vi "practica113b.vi"() -> ()   [LabVIEW 2016]
uses:
  <vilib>/Native 3D Graph/xcontrol/3DPC_SurfacePlot.xctl
panel:
  in  "Sz":dbl(slide) scale=0.0..10.0
  in  "s3":dbl(slide) max=1.4285714285714286 scale=0.0..3.4693877551020407
  in  "xy":dbl(knob) scale=0.0..360.0
  in  "xy2":dbl(knob) scale=-175.0..175.0
  out "3D Graph":refnum<class "Base Datatype.lvclass">[](xcontrol)
  in  "s1":dbl
  in  "s2":dbl
  in  "stop":bool
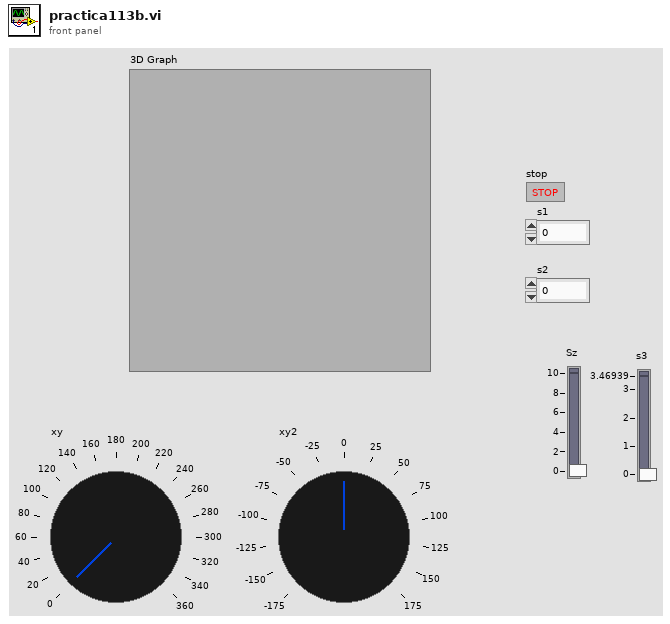
[diagram p1: front panel]
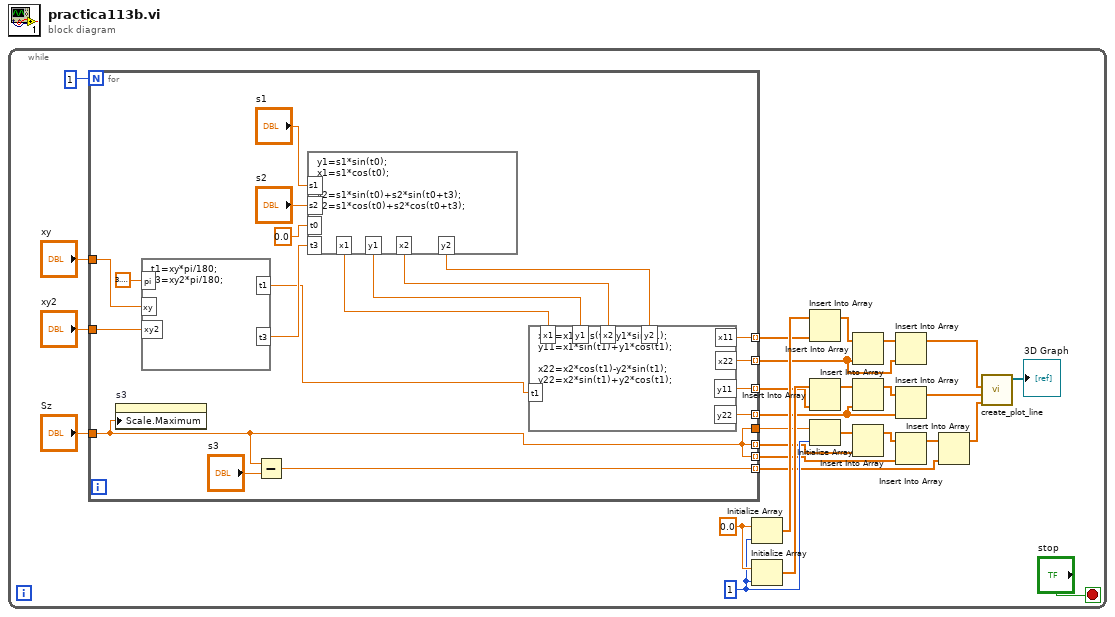
[diagram p0: block diagram]
diagram:
  n1 = while {
    stop <- "stop" stop-if-true
    w18 = 0.0
    w16 = 1 ("dimension size")
    n2 = for {
      N: 1 -> [_]
      tunnel: "xy" -> [w46]
      tunnel: "xy2" -> [w45]
      tunnel: [w33] -> w7 mode=indexing
      tunnel: [w35] -> w17 mode=indexing
      tunnel: [w32] -> w8 mode=indexing
      tunnel: [w34] -> w15 mode=indexing
      tunnel: [w29] -> w14 mode=indexing
      tunnel: [w29] -> w13 mode=indexing
      tunnel: [w30] -> w9 mode=indexing
      tunnel: "Sz" -> [w29]
      tunnel: [w29] -> w1
      n3 = property on="s3" class="Slide (strict)"("Scale.Maximum"=w29) -> ()  [unwired: 2 in, 2 out]
      n4 = formula code="t1=xy*pi/180;\nt3=xy2*pi/180;"("pi"=3.141592653589793, "xy"=w46, "xy2"=w45) -> ("t1"=w38:dbl, "t3"=w43:dbl)
      n5 = Subtract(x=w29, y="s3") -> (x-y=w30:dbl)
      n6 = formula code="y1=s1*sin(t0);\nx1=s1*cos(t0);\n\ny2=s1*sin(t0)+s2*sin(t0+t3);\nx2=s1*cos(t0)+s2*cos(t0+t3);"("t0"=0.0 ("input variable"), "s1"="s1", "s2"="s2", "t3"=w43) -> ("y1"=w39:dbl, "x1"=w40:dbl, "y2"=w36:dbl, "x2"=w37:dbl)
      n7 = formula code="x11=x1*cos(t1)-y1*sin(t1);\ny11=x1*sin(t1)+y1*cos(t1);\n\nx22=x2*cos(t1)-y2*sin(t1);\ny22=x2*sin(t1)+y2*cos(t1);"("x1"=w40, "y1"=w39, "t1"=w38, "x2"=w37, "y2"=w36) -> ("y11"=w34:dbl, "x11"=w35:dbl, "y22"=w32:dbl, "x22"=w33:dbl)
    }
    n8 = Initialize Array(w18, w16) -> (w22:dbl[])
    n9 = Initialize Array(w18, w16) -> (w23:dbl[])
    n10 = Insert Into Array(array=w22, new element=w17) -> (w19:dbl[])  [unwired: 1 in]
    n11 = Insert Into Array(array=w23, new element=w15) -> (w20:dbl[])  [unwired: 1 in]
    n12 = Initialize Array(w1, w16) -> (w3:dbl[])
    n13 = Insert Into Array(array=w19, new element=w7) -> (w12:dbl[])  [unwired: 1 in]
    n14 = Insert Into Array(array=w20, new element=w8) -> (w11:dbl[])  [unwired: 1 in]
    n15 = Insert Into Array(array=w3, new element=w14) -> (w21:dbl[])  [unwired: 1 in]
    n16 = Insert Into Array(array=w12, new element=w7) -> (w6:dbl[])  [unwired: 1 in]
    n17 = Insert Into Array(array=w11, new element=w8) -> (w5:dbl[])  [unwired: 1 in]
    n18 = Insert Into Array(array=w21, new element=w13) -> (w10:dbl[])  [unwired: 1 in]
    n19 = Insert Into Array(array=w10, new element=w9) -> (w4:dbl[])  [unwired: 1 in]
    n20 = call <vilib>:"create_plot_line.vi"("z vector"=w4, "y vector"=w5, "x vector"=w6) -> ("plots out"=→"3D Graph":refnum<class "Base Datatype.lvclass">[])  [unwired: 2 in, 6 out]
  }
